vi "Check Expected Terminal and Message Counts.vi"(5 "expected messages":i32=15, 7 "expected terminals":T1[](array[typedef])=[0], 8 "error in":errorcluster, 10 "custom device":T2 format="%.0x", 11 "Create Execution Unit in":refnum<class "Create Execution Unit.lvclass">) -> (0 "error out":errorcluster, 2 "custom device out":T2 format="%.0x", 3 "Create Execution Unit out":refnum<class "Create Execution Unit.lvclass">)   [LabVIEW 2020, in "Create Execution Unit.lvclass"]
uses:
  Create Execution Unit.lvclass
  Scripting/AIM MIL-STD-1553 Scripting.lvlib
  <vilib>/NI VeriStand/Custom Device API/Custom Device Item Ref.ctl
  <vilib>/NI VeriStand/Custom Device API/Custom Device API.lvlib
  Shared/Address.ctl
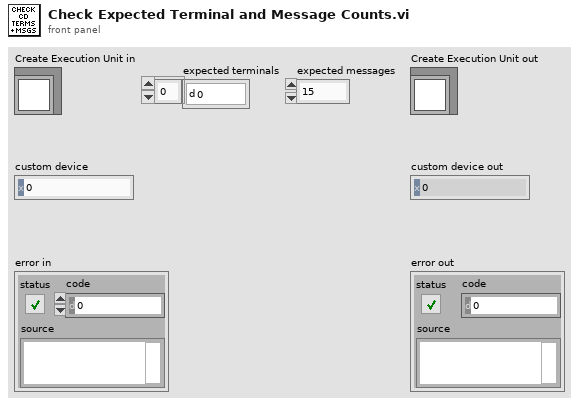
[diagram p1: front panel]
types:
  T1 = typedef "Address.ctl" = u16
  T2 = typedef "Custom Device API.lvlib/Custom Device Item Ref.ctl" = u64
  T3 = typedef "BIU Configuration.ctl" = cluster{"HW channel":u16, "terminal addresses":T1[], "terminal names":string[], "major frames":T4[], "minor frames":T5[], "acyclic frames":T6[], "messages":T7[]}
  T4 = typedef "Major Frame Definition.ctl" = cluster{"name":string, "minor frames":string[]}
  T5 = typedef "Minor Frame Definition.ctl" = cluster{"name":string, "messages":string[]}
  T6 = typedef "Acyclic Frame Definition.ctl" = cluster{"name":string, "messages":string[]}
  T7 = typedef "Message Definition.ctl" = cluster{"name":string, "message type":T8, "endpoint Tx":T9, "endpoint Rx":T9, "create timestamp channel":bool, "mode code":u16, "number of words":u16, "parameters":cluster{"name":string, "default value":dbl, "unit":string, "parameter definition":T10}[]}
  T8 = typedef "Message Type.ctl" = string
  T9 = typedef "Terminal Endpoint.ctl" = cluster{"terminal address":T1, "subaddress":T1}
  T10 = typedef "Parameter Definition.ctl" = cluster{"start index":i32, "size (bits)":i32, "encoding":enum16{"BNR", "BCD", "Discrete"}, "signed":bool, "multiplier":dbl, "offset":dbl}
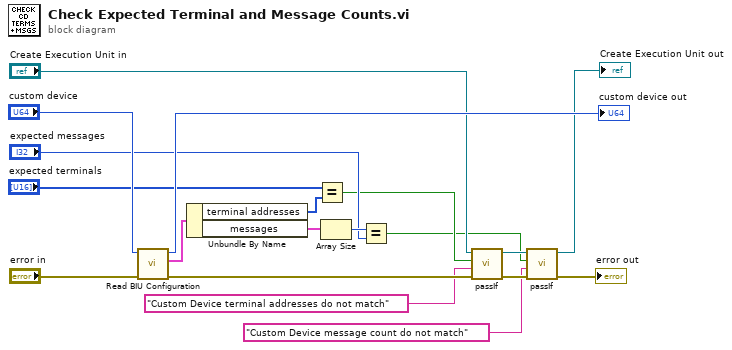
[diagram p0: block diagram]
diagram:
  n1 = call "Read BIU Configuration.vi"("error in"="error in", "custom device"="custom device") -> ("error out"=w9:errorcluster, "biu configuration"=w16:T3, "custom device out"=→"custom device out":T2)  [unwired: 7 in]
  n2 = Unbundle By Name(w16) -> ("terminal addresses"=w11:T1[], "messages"=w13:T7[])
  n3 = Equal?(x="expected terminals", y=w11) -> (x = y?=w7:bool)
  n4 = Array Size(array=w13) -> (size(s)=w15:i32)
  n5 = Equal?(x=w15, y="expected messages") -> (x = y?=w2:bool)
  n6 = call-dynamic "passIf.vi"("error in (no error)"=w9, "message (\"\")"="Custom Device terminal addresses do not match" ("message (\"\")"), "pass"=w7, "TestCase in"="Create Execution Unit in") -> ("error out"=w6:errorcluster, "TestCase out"=w5:refnum<class "Create Execution Unit.lvclass">)  [unwired: 6 in]
  n7 = call-dynamic "passIf.vi"("error in (no error)"=w6, "message (\"\")"="Custom Device message count do not match" ("message (\"\")"), "pass"=w2, "TestCase in"=w5) -> ("error out"=→"error out":errorcluster, "TestCase out"=→"Create Execution Unit out":refnum<class "Create Execution Unit.lvclass">)  [unwired: 6 in]
